vi "Test Test Finder Find Correct Number of Methods in Suite.vi"(8 "error in (no error)":errorcluster, 11 "Test Finder In":refnum<class "Test Finder.lvclass">) -> (0 "error out":errorcluster, 3 "Test Finder Out":refnum<class "Test Finder.lvclass">)   [LabVIEW 2020, in "LUnit Tests.lvlib" / "Test Finder.lvclass"]
uses:
  Test Finder.lvclass
  C:/Program Files (x86)/National Instruments/LabVIEW 2020/vi.lib/Asteme/LUnit/Test Case.lvclass
  Test Dummys/Descending Test Test Case/Descending Test Test Case.lvclass
  C:/Users/anton/Documents/GitHub/LUnit/source/Framework/Test Case/LUnit Test Case.lvclass
  source/Framework/Test Suite/LUnit Test Suite.lvclass
  Test Finder.lvclass/Test Finder.ctl
  source/Framework/Test Suite/LUnit Test Suite.lvclass/LUnit Test Suite.ctl
  source/Framework/Test Case/LUnit Test Case.lvclass/LUnit Test Case.ctl
  source/Framework/Helper Classes/Test Finder/Test Finder.lvclass/Test Finder.ctl
  <vilib>/Asteme/LUnit/Test Case.lvclass/Test Case.ctl
  <vilib>/Asteme/LUnit/LUnit Assertion Result.lvclass/LUnit Assertion Result.ctl
  <vilib>/Asteme/LUnit/LUnit Test Case Result.lvclass/LUnit Test Case Result.ctl
  <vilib>/Asteme/LUnit/LUnit Method Result.lvclass/LUnit Method Result.ctl
  source/Framework/Test Case/Public/Accessors/Read Enabled Test Methods.vi
  <vilib>/Asteme/LUnit/Palette/Pass.vi
  <vilib>/Asteme/LUnit/Palette/Fail.vi
  <vilib>/Asteme/LUnit/Variant to string.vi
  <vilib>/Asteme/LUnit/Set Assertion Type.vi
  <vilib>/Asteme/LUnit/Add test result.vi
  <vilib>/Asteme/LUnit/LUnit Write Passed.vi
  <vilib>/Asteme/LUnit/LUnit Write Message.vi
  <vilib>/Asteme/LUnit/LUnit Write Description.vi
  <vilib>/Asteme/LUnit/LUnit Write Assertion Type.vi
  <vilib>/Asteme/LUnit/LUnit Record Assertion Result.vi
  <vilib>/Asteme/LUnit/LUnit Aggregate Assertion Results.vi
  <vilib>/Asteme/LUnit/Assertion Result/LUnit Read Status.vi
  <vilib>/Asteme/LUnit/LUnit Read Message.vi
  <vilib>/Asteme/LUnit/LUnit Read Description.vi
  <vilib>/Asteme/LUnit/Method Result/LUnit Merge Status.vi
  <vilib>/Asteme/LUnit/LUnit Concatenate result strings.vi
  source/Framework/Helper Classes/Test Finder/Public/Accessors/Read Test Method Names.vi
  <vilib>/Utility/Data Type/Get Type Information.vi
  <vilib>/Utility/LVClass/Get LV Class Name.vi
  source/Framework/Helper Classes/Test Finder/Test Finder.lvclass
  <vilib>/Asteme/LUnit/LUnit Assertion Result.lvclass
  <vilib>/Asteme/LUnit/Test Case.lvclass
  Test Dummys/Test Test Case/Test Test Case.lvclass
  C:/Users/anton/Documents/GitHub/LUnit/tests/Test Dummys/Test Test Case/Test Test Case.lvclass
  C:/Users/anton/Documents/GitHub/LUnit/tests/Test Dummys/Descending Test Test Case/Descending Test Test Case.lvclass
  C:/Users/anton/Documents/GitHub/LUnit/tests/Test Finder/Test Finder.lvclass
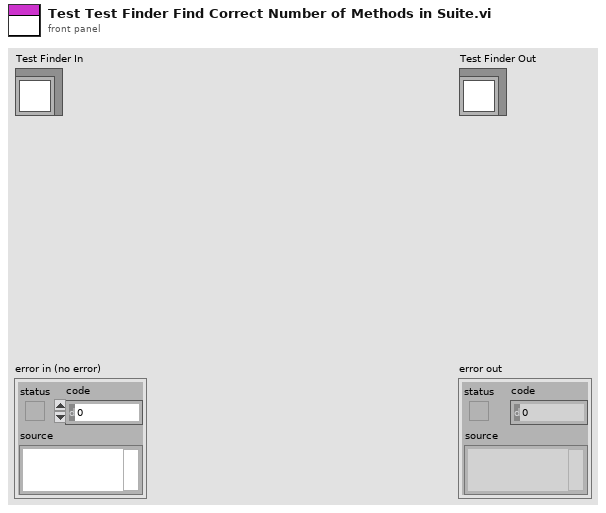
[diagram p1: front panel]
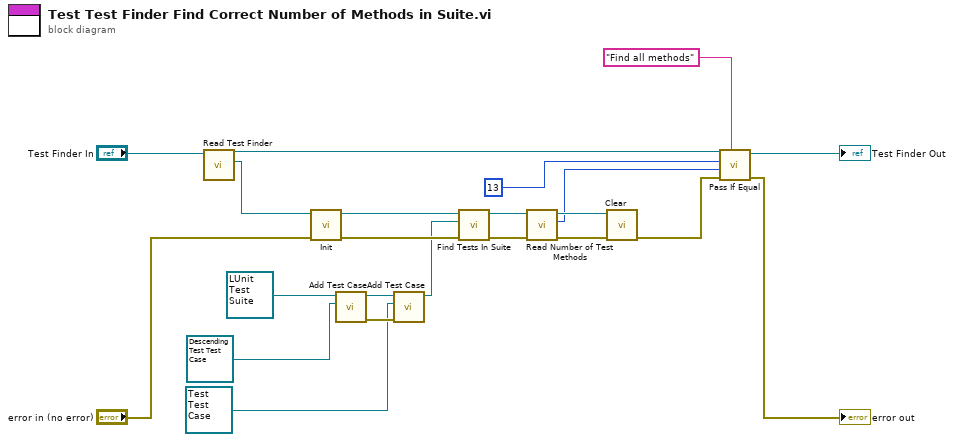
[diagram p0: block diagram]
diagram:
  n1 = call "Read Test Finder.vi"("Test Finder In"="Test Finder In") -> ("Test Finder.lvclass"=w21:refnum<class "Test Finder.lvclass">, "Test Finder Out"=w13:refnum<class "Test Finder.lvclass">)  [unwired: 8 in, 1 out]
  n2 = call-dynamic "Init.vi"("error in (no error)"="error in (no error)", "Test Finder in"=w21) -> ("error out"=w19:errorcluster, "Test Finder out"=w20:refnum<class "Test Finder.lvclass">)  [unwired: 8 in]
  n3 = call "Add Test Case.vi"("Test Case to add"=refnum<class "Descending Test Test Case.lvclass"> refnum ("Descending Test Test Case.lvclass"), "Test Suite In"=refnum<class "LUnit Test Suite.lvclass"> refnum) -> ("error out"=w5:errorcluster, "Test Suite Out"=w4:refnum<class "LUnit Test Suite.lvclass">)  [unwired: 8 in]
  n4 = call "Add Test Case.vi"("error in (no error)"=w5, "Test Case to add"=refnum<class "Test Test Case.lvclass"> refnum ("Test Test Case.lvclass"), "Test Suite In"=w4) -> ("Test Suite Out"=w3:refnum<class "LUnit Test Suite.lvclass">)  [unwired: 7 in, 1 out]
  n5 = call "Find Tests In Suite.vi"("error in (no error)"=w19, "Test Suite"=w3, "Test Finder In"=w20) -> ("error out"=w16:errorcluster, "Test Finder Out"=w18:refnum<class "Test Finder.lvclass">)  [unwired: 7 in]
  n6 = call "Read Number of Test Methods.vi"("error in (no error)"=w16, "Test Finder In"=w18) -> ("error out"=w15:errorcluster, "Number of Test Methods found"=w7:i32, "Test Finder Out"=w17:refnum<class "Test Finder.lvclass">)  [unwired: 7 in]
  n7 = call "Clear.vi"("error in (no error)"=w15, "Test Finder in"=w17) -> ("error out"=w11:errorcluster)  [unwired: 8 in, 1 out]
  n8 = call <vilib>:"Pass If Equal.vi"("Description"="Find all methods", "error in (no error)"=w11, "Actual"=w7, "Expected"=13 ("x"), "LUnit Test Case In"=w13) -> ("error out"=→"error out":errorcluster, "LUnit Test Case Out"=→"Test Finder Out":refnum<class "Test Finder.lvclass">)  [unwired: 5 in]
